vi "remote.Read Dev.Properties.vi"(8 "error in (no error)":errorcluster, 11 "SLSC Remote in":refnum<class "SLSC Remote.lvclass">) -> (0 "error out":errorcluster, 2 "Dev.Properties":refnum<k21>[](array[refnum]), 3 "SLSC Remote out":refnum<class "SLSC Remote.lvclass">)   [LabVIEW 2016, in "SLSC Interfaces.lvlib" / "SLSC Remote.lvclass"]
uses:
  SLSC Remote.lvclass
  <vilib>/NI/JSON Support for LabVIEW/JSON Data Classes/JSON Helper/JSON Helper.lvclass
  <vilib>/NI/JSON Support for LabVIEW/JSON Data Classes/JSON Array/JSON Array.lvclass
  <vilib>/NI/JSON Support for LabVIEW/JSON Data Classes/JSON Array/Index Array (String Value).vi
  <vilib>/NI/JSON Support for LabVIEW/JSON Data Classes/JSON Helper/To More Specific Type (Array).vi
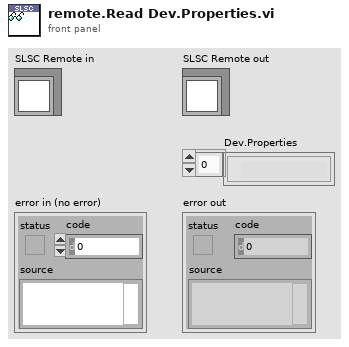
[diagram p1: front panel]
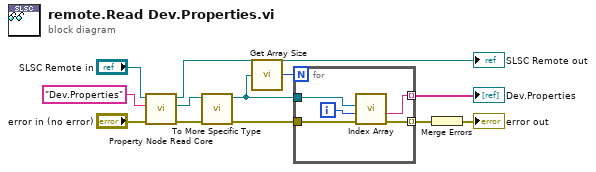
[diagram p0: block diagram]
diagram:
  n1 = call "Property Node Read Core.vi"("error in (no error)"="error in (no error)", "property"="Dev.Properties", "SLSC Remote in"="SLSC Remote in") -> ("error out"=w3:errorcluster, "value"=w4:refnum<class "JSON Null.lvclass">, "SLSC Remote out"=→"SLSC Remote out":refnum<class "SLSC Remote.lvclass">)  [unwired: 6 in]
  n2 = call-poly <vilib>:"To More Specific Type.vi"("error in (no error)"=w3, "JSON Datatype in"=w4) -> ("error out"=w8:errorcluster, "JSON Datatype out"=w7:refnum<class "JSON Array.lvclass">)  [unwired: 8 in]
  n3 = call <vilib>:"Get Array Size.vi"("JSON Array in"=w7) -> ("size(s)"=w6:i32)
  n4 = for {
    N: w6 -> [_]
    tunnel: w7 -> [w16]
    tunnel: w8 -> [w15]
    tunnel: [w14] -> w5 mode=indexing
    tunnel: [w13] -> w1 mode=indexing
    i -> [w17]
    n5 = call-poly <vilib>:"Index Array.vi"("error in (no error)"=w15, "index"=w17, "JSON Array in"=w16) -> ("error out"=w14:errorcluster, "String"=w13:string)  [unwired: 7 in]
  }
  "Dev.Properties" <- w1
  n6 = Merge Errors(w5) -> (→"error out":errorcluster)
